vi "Cycle Average and RMS.vi"   [LabVIEW 2020, in "NI_MAPro.lvlib"]
doc: "Returns the average and RMS levels of a selected cycle of a periodic waveform or an array of periodic waveforms. Wire data to the <B>signal in</B> input to determine the polymorphic instance to use or manually select the instance."
uses:
  NI_MAPro.lvlib
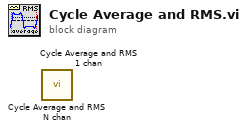
[diagram p0: block diagram]
diagram:
  n1 = call "Cycle Average and RMS N chan.vi"() -> ()  [unwired: 8 in, 4 out]
  n2 = call "Cycle Average and RMS 1 chan.vi"() -> ()  [unwired: 8 in, 4 out]
